vi "32 RMS.vi"() -> ()   [LabVIEW 2017]
panel:
  in  "length":dbl=60.0 format="%#_13g"
  in  "min bin":i32=30
  out "index":i32=31
  out "TDC 32 RMS":dbl[](graph)=[0.0, 4.495188001799701, 4.047951877770932, 3.7983006028212425, 4.489575213445057, 3.9309524944114287, 3.707770991642911, 3.9095038865717506, 5.029793785599916, 4.93349045269778, 5.280716960843466, 4.009117287079073, 4.753090086741872, 4.964068571572402, 5.792493126476514, 4.636862858134927, 5.324844590529911, 5.965341293736383, 5.55451644090397, 5.613124265523868, 4.113119233346008, 8.790736111740454, 3.87163174955266, 4.47852946608946, 4.676704953615258, 5.592120403000107, 5.167516606870649, 5.2288050691508, 4.22997766658757, 5.478411410871065, 4.8903119015295164, 3.9897787304605288]
  out "Array":dbl[](array[numeric])=[0.0, 4.495188001799701, 4.047951877770932, 3.7983006028212425, 4.489575213445057, 3.9309524944114287, 3.707770991642911, 3.9095038865717506, 5.029793785599916, 4.93349045269778, 5.280716960843466, 4.009117287079073, 4.753090086741872, 4.964068571572402, 5.792493126476514, 4.636862858134927, 5.324844590529911, 5.965341293736383, 5.55451644090397, 5.613124265523868, 4.113119233346008, 8.790736111740454, 3.87163174955266, 4.47852946608946, 4.676704953615258, 5.592120403000107, 5.167516606870649, 5.2288050691508, 4.22997766658757, 5.478411410871065, 4.8903119015295164, 3.9897787304605288]
  in  "base channel":i32
  in  "file path (dialog if empty)":path=path "F:/UserData/My Documents/WeChat Files/wxid_g1lgpn15cu3722/FileStorage/File/2023-01/test_20230109_030257.csv"
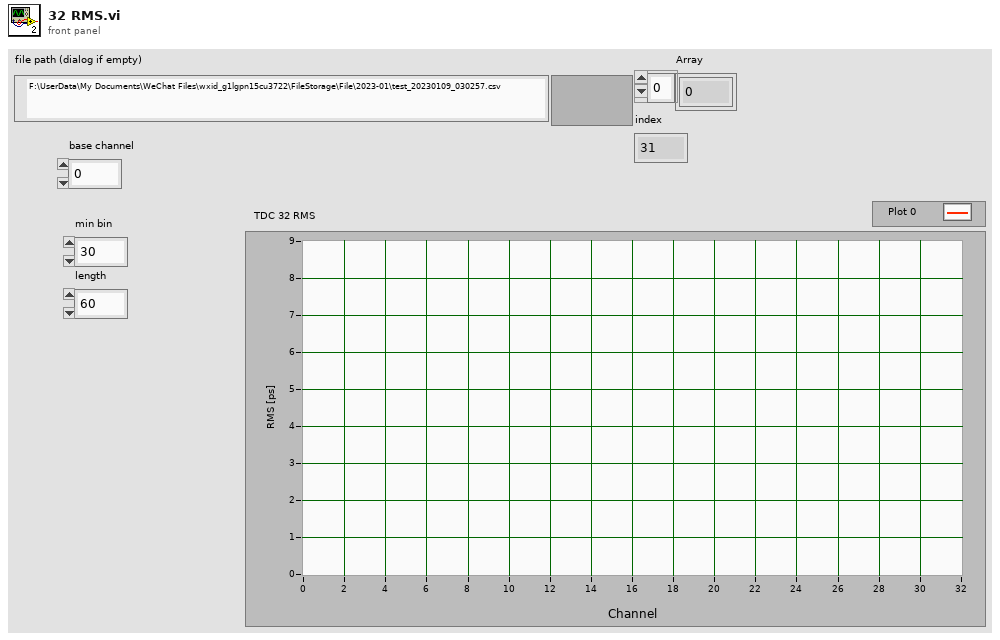
[diagram p1: front panel]
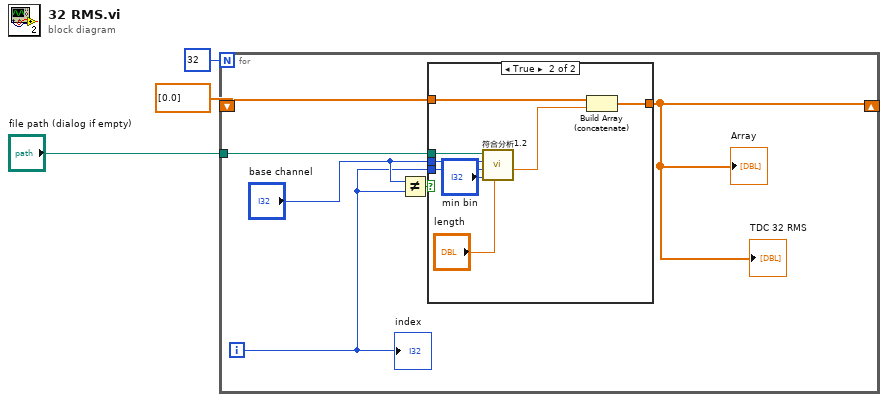
[diagram p0: block diagram]
diagram:
  n1 = for {
    N: 32 -> [_]
    tunnel: "file path (dialog if empty)" -> [w9]
    shift-right: [w4] -> _
    shift-left: dbl[] [0.0] -> [w5]
    i -> [w6]
    n2 = Not Equal?(x="base channel", y=w6) -> (x != y?=w8:bool)
    n3 = case shown="True" w8 {
      tunnel: w9 -> [_ w18]
      tunnel: "base channel" -> [_ w17]
      tunnel: w6 -> [_ w16]
      tunnel: [w10 w15] -> w4
      tunnel: w5 -> [w10 w14]
      frame False {
      }
      frame True {
        n4 = call "符合分析1.2.vi"("length"="length", "min bin"="min bin", "通道B"=w16, "通道A"=w17, "file path (dialog if empty)"=w18) -> ("Fitting RMS"=w13:dbl)  [unwired: 5 in, 1 out]
        n5 = Build Array (concatenate)(w14, w13) -> (w15:dbl[])
      }
    }
    "Array" <- w4
    "TDC 32 RMS" <- w4
    "index" <- w6
  }
